vi "PathtoDirPath.vi"(1 "Path":path) -> (0 "Path out":path)   [LabVIEW 2013]
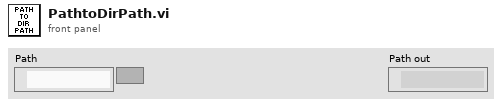
[diagram p1: front panel]
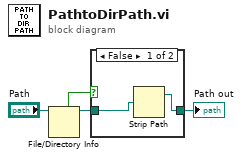
[diagram p0: block diagram]
diagram:
  n1 = File/Directory Info(path="Path") -> (path out=w3:path, directory=w4:bool)  [unwired: 1 in, 5 out]
  n2 = case shown="False" w4 {
    tunnel: w3 -> [w6 w7]
    tunnel: [w5 w7] -> w1
    frame False {
      n3 = Strip Path(path=w6) -> (stripped path=w5:path)  [unwired: 1 out]
    }
    frame True {
    }
  }
  "Path out" <- w1
